vi "Ctor.vi"(8 "error in (no error)":errorcluster, 11 "TCP Server in":refnum<class "TCP Server.lvclass">) -> (0 "error out":errorcluster, 3 "TCP Server out":refnum<class "TCP Server.lvclass">)   [LabVIEW 2020, in "Stream-TCP.lvlib" / "TCP Server.lvclass"]
uses:
  TCP Server.lvclass
  Ref Data.ctl
  TCP Client/TCP Client.lvclass
  Listener Result.ctl
  Listener Status.ctl
  TCP Server.lvclass/TCP Server.ctl
  <vilib>/IlluminatedG/lv-stream/Endpoint/Endpoint.lvclass
  Stream-TCP.lvlib
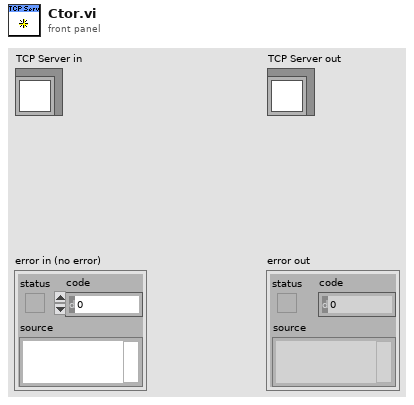
[diagram p1: front panel]
types:
  T1 = typedef "Stream-TCP.lvlib/Listener Result.ctl" = cluster{"Status":T2, "Client":refnum<class "TCP Client.lvclass">, "Ack Notifier":refnum<notifier>}
  T2 = typedef "Stream-TCP.lvlib/Listener Status.ctl" = enum16{"Successful", "Unsuccessful"}
  T3 = typedef "Stream-TCP.lvlib/TCP Server.lvclass/Ref Data.ctl" = cluster{"Listener":refnum<k5>, "Clients":refnum<class "TCP Client.lvclass">[], "Server Loop":bool}
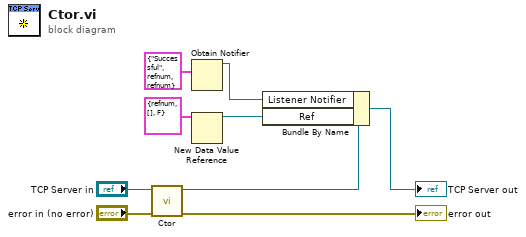
[diagram p0: block diagram]
diagram:
  n1 = call-parent "Ctor.vi"("error in (no error)"="error in (no error)", "Endpoint in"="TCP Server in") -> ("error out"=→"error out":errorcluster, "Endpoint out"=w9:refnum<class "TCP Server.lvclass">)  [unwired: 8 in]
  n2 = Obtain Notifier(notification data type=T1 {"Status"=enum."Successful", "Client"=refnum, "Ack Notifier"=refnum} ("Result")) -> (notifier out=w2:refnum<notifier>)  [unwired: 3 in, 2 out]
  n3 = New Data Value Reference(data value=T3 {"Listener"=refnum, "Clients"=[], "Server Loop"=FALSE} ("Ref Data")) -> (data value reference=w3:refnum<data-value>)  [unwired: 1 in, 1 out]
  n4 = Bundle By Name(cluster=w9, "Listener Notifier"=w2, "Ref"=w3) -> (→"TCP Server out":refnum<class "TCP Server.lvclass">)
